vi "Wizard Check Database.vi"(8 "error in":errorcluster, 11 "Database Location":path) -> (0 "error out":errorcluster, 3 "Binding":bool)   [LabVIEW 2014]
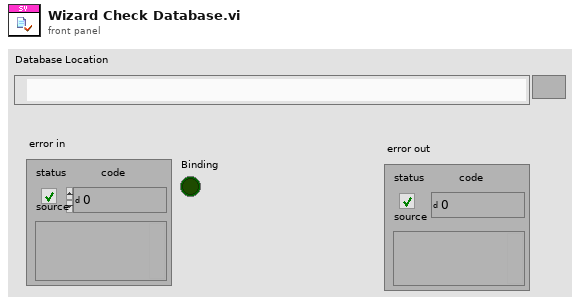
[diagram p1: front panel]
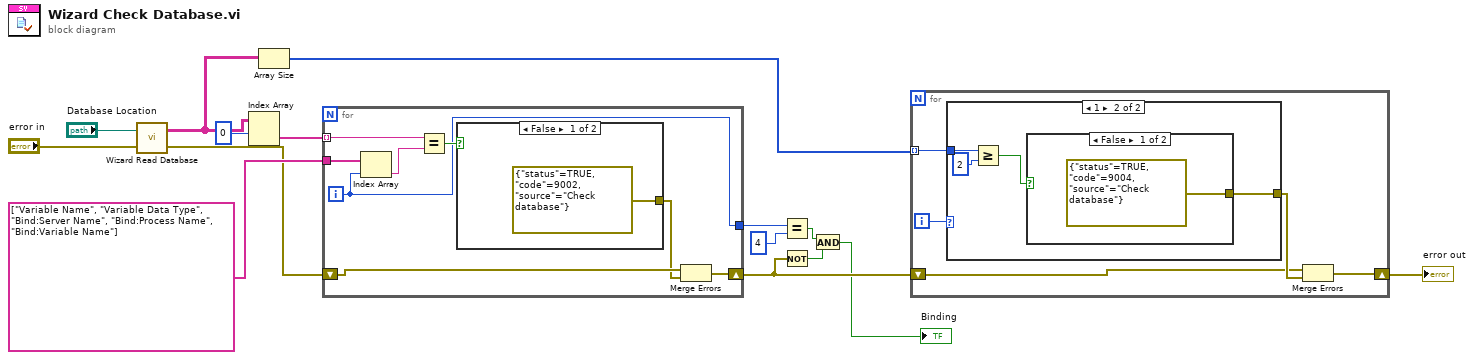
[diagram p0: block diagram]
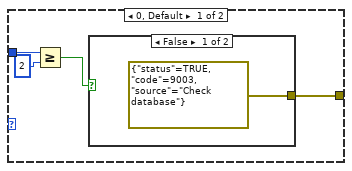
[diagram p2: hidden frame]
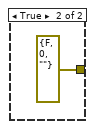
[diagram p3: hidden frame]
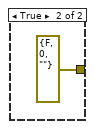
[diagram p4: hidden frame]
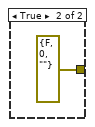
[diagram p5: hidden frame]
diagram:
  n1 = call "Wizard Read Database.vi"("error in (no error)"="error in", "Database Location"="Database Location") -> ("error out"=w10:errorcluster, "Database"=w9:string[][])
  n2 = Index Array(array=w9, index (row)=0) -> (element=w7:string[])  [unwired: 1 in]
  n3 = Array Size(array=w9) -> (size(s)=w14:i32[])
  n4 = for {
    tunnel: string[] ["Variable Name", "Variable Data Type", "Bind:Server Name", "Bind:Process Name", "Bind:Variable Name"] -> [w23]
    shift-right: [w20] -> w2
    shift-left: w10 -> [w18]
    tunnel: w7 -> [w19] mode=indexing
    tunnel: [w16] -> w6
    i -> [w16]
    n5 = Index Array(array=w23, index=w16) -> (element=w22:string)
    n6 = Equal?(x=w19, y=w22) -> (x = y?=w21:bool)
    n7 = case shown="False" w21 {
      tunnel: [errorcluster {"status"=TRUE, "code"=9002, "source"="Check database"} ("error constant") errorcluster {"status"=FALSE, "code"=0, "source"=""} ("error constant")] -> w17
      frame False {
      }
      frame True {
      }
    }
    n8 = Merge Errors(w18, w17) -> (w20:errorcluster)
  }
  n9 = Equal?(x=w6, y=4) -> (x = y?=w4:bool)
  n10 = Not(x=w2) -> (.not. x?=w3:bool)
  n11 = And(x=w4, y=w3) -> (x .and. y?=→"Binding":bool)
  n12 = for {
    shift-right: [w28] -> w13
    shift-left: w2 -> [w26]
    tunnel: w14 -> [w29] mode=indexing
    i -> [w30]
    n13 = case shown="1" w30 {
      tunnel: w29 -> [w34 w40]
      tunnel: [w31 w37] -> w27
      frame 0, Default {
        n14 = Greater Or Equal?(x=w34, y=2) -> (x >= y?=w32:bool)
        n15 = case shown="False" w32 {
          tunnel: [errorcluster {"status"=TRUE, "code"=9003, "source"="Check database"} ("error constant") errorcluster {"status"=FALSE, "code"=0, "source"=""} ("error constant")] -> w31
          frame False {
          }
          frame True {
          }
        }
      }
      frame 1 {
        n16 = Greater Or Equal?(x=w40, y=2) -> (x >= y?=w38:bool)
        n17 = case shown="False" w38 {
          tunnel: [errorcluster {"status"=TRUE, "code"=9004, "source"="Check database"} ("error constant") errorcluster {"status"=FALSE, "code"=0, "source"=""} ("error constant")] -> w37
          frame False {
          }
          frame True {
          }
        }
      }
    }
    n18 = Merge Errors(w26, w27) -> (w28:errorcluster)
  }
  "error out" <- w13
